vi "连接配置对话框.vi"() -> (14 "check？":bool)   [LabVIEW 2016, in "PLC.lvlib"]
uses:
  PLC.lvlib
panel:
  in  "取消":bool
  in  "确定":bool
  in  "连接配置":T1={"连接类型"=enum."TCP", "串口"="COM3", "IP"="192.168.1.200", "PORT"=502}
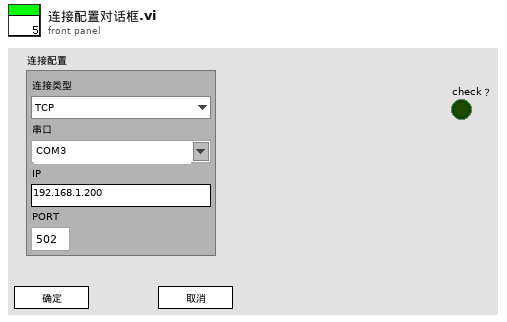
[diagram p1: front panel]
types:
  T1 = cluster{"连接类型":enum16{"串口", "TCP"}, "串口":string, "IP":string, "PORT":u16}
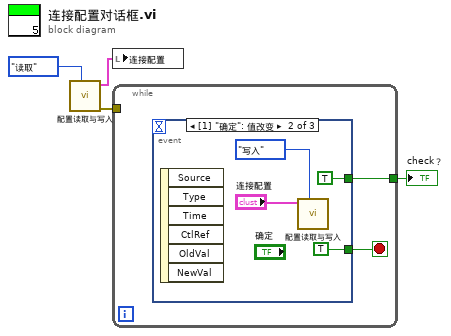
[diagram p0: block diagram]
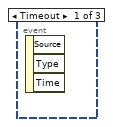
[diagram p2: hidden frame]
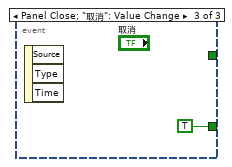
[diagram p3: hidden frame]
diagram:
  n1 = call "配置读取与写入.vi"("功能"=enum16{"读取", "写入"}."读取") -> ("error out"=w2:errorcluster, "连接配置 2"=w3:T1)  [unwired: 9 in]
  n2 = local write "连接配置"(w3) -> ()
  n3 = while {
    tunnel: w2 -> [_]
    tunnel: [w5] -> w1
    stop <- w6 stop-if-true
    n4 = event shown="[1] \"确定\": 值改变" {
      selector: _ -> [_ _ _]
      dyn-events: _ -> [_ _ _]
      timeout: _ -> [_ _ _]
      tunnel: [_ TRUE TRUE] -> w6
      tunnel: [_ TRUE _] -> w5
      event Timeout {
        n5 = event-data() -> ()  [unwired: 1 in, 3 out]
      }
      event "确定": Value Change {
        n6 = event-data() -> ()  [unwired: 1 in, 6 out]
        n7 = call "配置读取与写入.vi"("功能"=enum16{"读取", "写入"}."写入", "连接配置"="连接配置") -> ()  [unwired: 8 in, 2 out]
      }
      event Panel Close; "取消": Value Change {
        n8 = event-data() -> ()  [unwired: 1 in, 3 out]
      }
    }
  }
  "check？" <- w1
